vi "Get AppData Directory.vi"(8 "Error In":errorcluster) -> (0 "Error Out":errorcluster, 2 "Folder exists?":bool, 3 "Folder path":path)   [LabVIEW 2020]
doc: "Get the AppData folder from the regstry database.\nGives the Folder path and if it exists"
uses:
  <vilib>/registry/registry.llb/Registry RtKey.ctl
  <vilib>/registry/registry.llb/Read Registry Value Simple STR.vi
panel:
  out "number":dbl
  out "Operating System:Version Number":string
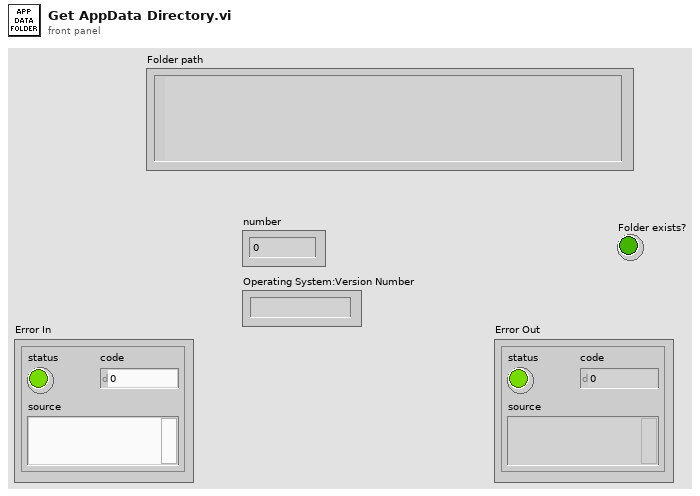
[diagram p1: front panel]
types:
  T1 = typedef "Registry RtKey.ctl" = enum32{"HKEY_CLASSES_ROOT", "HKEY_CURRENT_USER", "HKEY_LOCAL_MACHINE", "HKEY_USERS", "HKEY_PERFORMANCE_DATA", "HKEY_CURRENT_CONFIG", "HKEY_DYN_DATA"}
  T2 = typedef "Registry refnum.ctl" = refnum<k1>
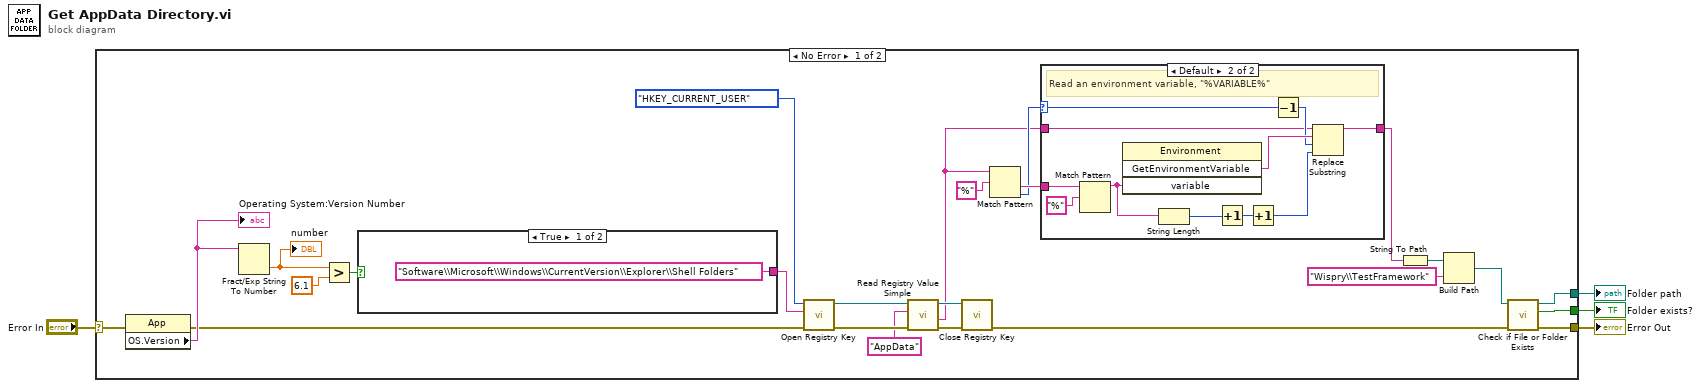
[diagram p0: block diagram]
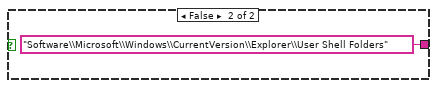
[diagram p3: hidden frame]
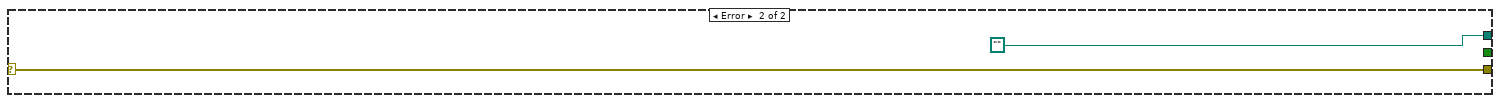
[diagram p4: hidden frame]
diagram:
  n1 = case shown="No Error" "Error In" {
    selector: "Error In" -> [w12 w45]
    tunnel: [w18 path ""] -> w3
    tunnel: [w17 _] -> w2
    tunnel: [w16 w45] -> w1
    frame No Error {
      n2 = property class="App"(error in=w12) -> (error out=w11:errorcluster, "OS.Version"=w14:string)  [unwired: 1 in, 1 out]
      "Operating System:Version Number" <- w14
      n3 = Fract/Exp String To Number(string=w14) -> (number=w15:dbl)  [unwired: 3 in, 1 out]
      "number" <- w15
      n4 = Greater?(x=w15, y=6.1) -> (0:w10:bool)
      n5 = case shown="True" w10 {
        tunnel: ["Software\\Microsoft\\Windows\\CurrentVersion\\Explorer\\Shell Folders" ("subkey") "Software\\Microsoft\\Windows\\CurrentVersion\\Explorer\\User Shell Folders" ("subkey")] -> w28
        frame True {
        }
        frame False {
        }
      }
      n6 = call <vilib>:"Open Registry Key.vi"("error in (no error)"=w11, "subkey"=w28, "root key (HKEY_LOCAL_MACHINE)"=Registry_RtKey."HKEY_CURRENT_USER") -> ("error out"=w27:errorcluster, "refnum out"=w26:T2)  [unwired: 7 in]
      n7 = call-poly <vilib>:"Read Registry Value Simple.vi"("error in (no error)"=w27, "value"="AppData", "refnum"=w26) -> ("error out"=w24:errorcluster, "String/Binary data"=w6:string, "refnum out"=w23:T2)  [unwired: 3 in, 1 out]
      n8 = call <vilib>:"Close Registry Key.vi"("error in (no error)"=w24, "refnum"=w23) -> ("error out"=w19:errorcluster)  [unwired: 5 in]
      n9 = Match Pattern(string=w6, regular expression="%") -> (after substring=w8:string, offset past match=w7:i32)  [unwired: 1 in, 2 out]
      n10 = case shown="Default" w7 {
        selector: w7 -> [_ w33]
        tunnel: w8 -> [_ w40]
        tunnel: w6 -> [w30 w32]
        tunnel: [w30 w31] -> w5
        frame -1 {
        }
        frame Default {
          # "Read an environment variable, \"%VARIABLE%\""
          n11 = Match Pattern(string=w40, regular expression="%") -> (before substring=w38:string)  [unwired: 1 in, 3 out]
          n12 = invoke class="Environment" method="GetEnvironmentVariable"("variable"=w38) -> ("GetEnvironmentVariable"=w39:string)  [unwired: 3 in, 3 out]
          n13 = String Length(string=w38) -> (length=w37:i32)
          n14 = Increment(x=w37) -> (x+1=w35:i32)
          n15 = Increment(x=w35) -> (x+1=w34:i32)
          n16 = Decrement(x=w33) -> (x-1=w36:i32)
          n17 = Replace Substring(2:w34, 3:w36, 4:w39, 5:w32) -> (1:w31:string)  [unwired: 1 out]
        }
      }
      n18 = String To Path(string=w5) -> (path=w22:path)
      n19 = Build Path(base path=w22, name or relative path="Wispry\\TestFramework") -> (appended path=w20:path)
      n20 = call <vilib>:"Check if File or Folder Exists.vi"("error in (no error)"=w19, "path"=w20) -> ("error out"=w16:errorcluster, "file or folder exists?"=w17:bool, "dup path"=w18:path)  [unwired: 7 in]
    }
    frame Error {
    }
  }
  "Error Out" <- w1
  "Folder path" <- w3
  "Folder exists?" <- w2
